vi "Static1DArray.vi"() -> ()   [LabVIEW 2020]
uses:
  Passing.dll
panel:
  out "arg1 2":dbl[](array[numeric])
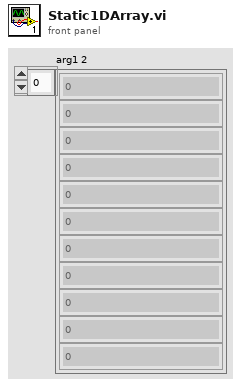
[diagram p1: front panel]
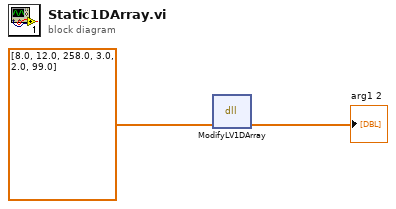
[diagram p0: block diagram]
diagram:
  n1 = dll-call lib="E:/Practice/Lv/dll/CppDllForLv/src/LV/Passing/Passing.dll" fn="ModifyLV1DArray"("arg1"=dbl[] [8.0, 12.0, 258.0, 3.0, 2.0, 99.0] ("arg1 2")) -> ("arg1"=→"arg1 2":dbl[])  [unwired: 4 in, 2 out]
